vi "AttackerPrepareKickEnemy.vi"(10 "Robot in":T1, 11 "balls":T6[](array[typedef])) -> (3 "Robot out":T1)   [LabVIEW 2018]
uses:
  Core/AI Ball.ctl
  Core/AI Robot.ctl
  Functions Enum.ctl
  AttackerStates.ctl
  Path Planning/RRT/PathDests.ctl
  Path Planning/RRT/PathDest.ctl
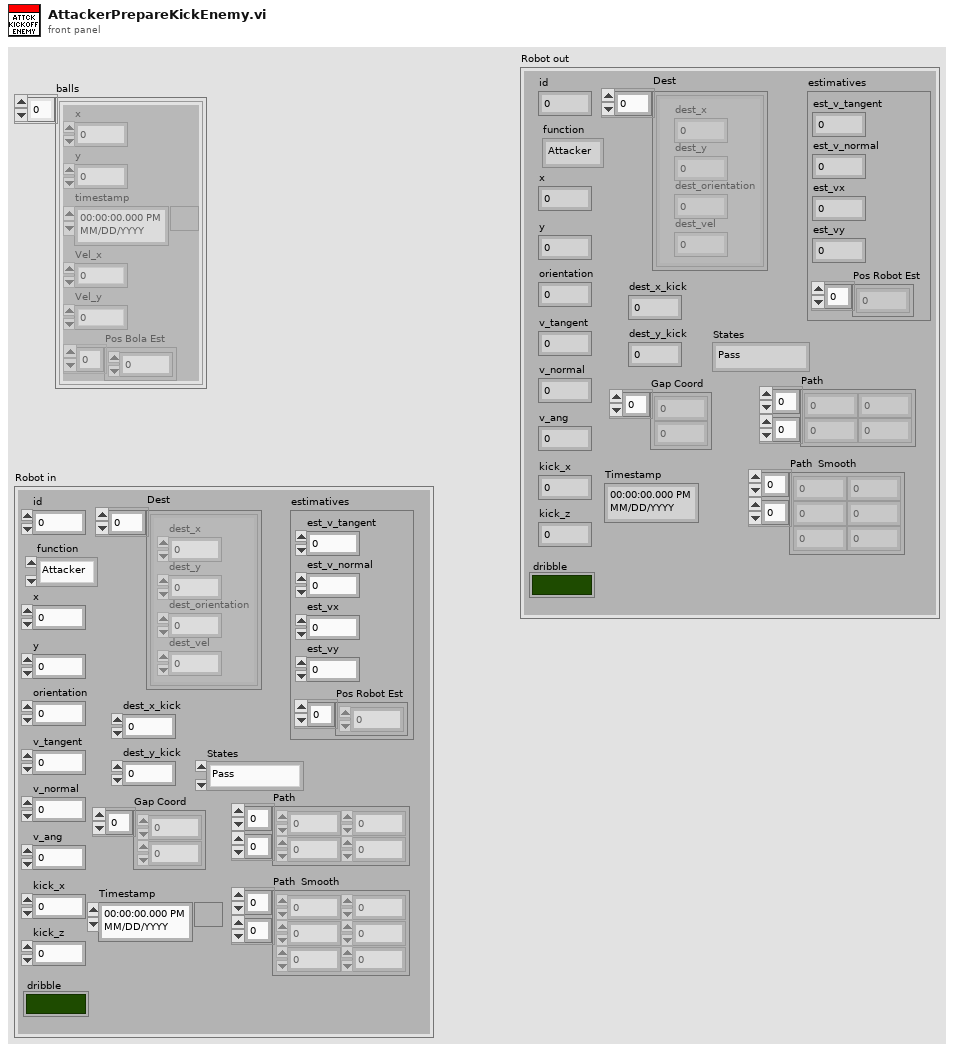
[diagram p1: front panel]
types:
  T1 = typedef "AI Robot.ctl" = cluster{"id":u32, "function":T2, "x":dbl, "y":dbl, "orientation":dbl, "v_tangent":dbl, "v_normal":dbl, "v_ang":dbl, "kick_x":dbl, "kick_z":dbl, "dribble":bool, "Timestamp":timestamp, "estimatives":cluster{"est_v_tangent":dbl, "est_v_normal":dbl, "est_vx":dbl, "est_vy":dbl, "Pos Robot Est":dbl[]}, "dest_x_kick":dbl, "dest_y_kick":dbl, "Gap Coord":dbl[], "States":T3, "Path ":dbl[][], "Path  Smooth":dbl[][], "Dest":T4}
  T2 = typedef "Functions Enum.ctl" = enum16{"Attacker", "Goalie", "Defender", "Striker", "Goto 0", "Dummy", "Kicker", "ZigZag"}
  T3 = typedef "AttackerStates.ctl" = enum16{"Pass", "GoToTangent", "BallGetting", "GoToKick", "Rotate anti-clockwise", "Rotate Clockwise", ""}
  T4 = typedef "PathDests.ctl" = T5[]
  T5 = typedef "PathDest.ctl" = cluster{"dest_x":dbl, "dest_y":dbl, "dest_orientation":dbl, "dest_vel":dbl}
  T6 = typedef "AI Ball.ctl" = cluster{"x":dbl, "y":dbl, "timestamp":timestamp, "Vel_x":dbl, "Vel_y":dbl, "Pos Bola Est":dbl[]}
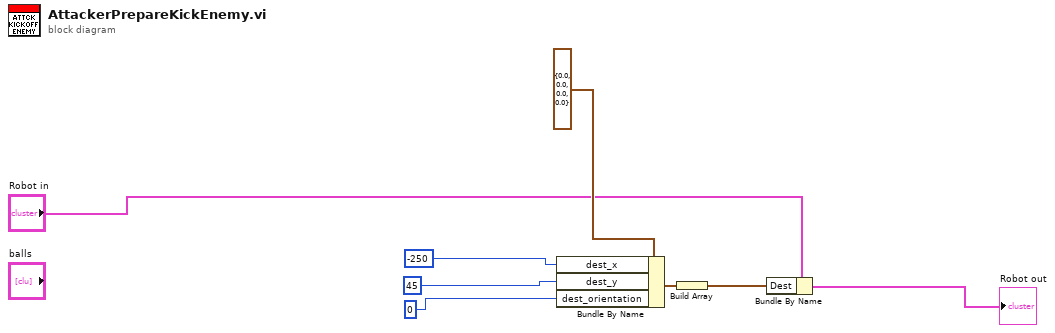
[diagram p0: block diagram]
diagram:
  n1 = Bundle By Name(cluster=T5 {"dest_x"=0.0, "dest_y"=0.0, "dest_orientation"=0.0, "dest_vel"=0.0} ("element"), "dest_x"=-250, "dest_y"=45, "dest_orientation"=0) -> (w7:T5)
  n2 = Build Array(w7) -> (w6:T5[])
  n3 = Bundle By Name(cluster="Robot in", "Dest"=w6) -> (→"Robot out":T1)
